vi "SubPanel_DataCollection_Rev11_v13.vi"(0 "DCPowerInformationClusterArray_Input":T6(array[cluster]), 1 "VISAPowerInfoInputArray":T5(array[cluster]), 2 "Run Data SubPanel Input":T4, 3 "RF Block Input Array":T1[](array[typedef]), 4 "Oscilloscope Info Array":T3(array[cluster]) {"vertical coupling" items=["AC", "DC", "Ground"]}, 5 "Plot Color Array":u32[](array[colorbox])=[16711686, 65351, 8978420, 14474240, 16139007, 16752640, 8958719, 16758973, 16777215, 46792, 11992992, 12961221, 16763690, 12600063, 16711835, 2953983, 40796, 13111296, 13352613, 9221011, 12964076, 12819897, 65442, 16776704, 14540253, 16740729, 10658047, 10813344, 16753521, 13413843, 8691115, 10339240, 14401205, 16746704, 7467519, 16775978, 13872558, 11387603, 13354405, 10420227, 13107364, 4060, 35208, 11817216, 7566080, 40796, 7539456, 2837073, 6372186, 7499083, 10648702, 16757152], 6 "New Run?":bool, 7 "error in":errorcluster) -> (20 "DCPowerInformationClusterArray_Output":T6(array[cluster]), 21 "VISAPowerInfoInputOutput":T5(array[cluster]), 22 "Run Data SubPanel Output":T4, 23 "RF Subpanel Output":T1[](array[typedef]), 24 "Oscilloscope Info Array Output":T3(array[cluster]) {"vertical coupling" items=["AC", "DC", "Ground"]}, 25 "Reinitialize?":bool, 26 "Data Was Collected?":bool, 27 "error out":errorcluster)   [LabVIEW 2019]
uses:
  Controls/DataBlockControl.ctl
  Controls/QueueDataControl_V3.ctl
  <vilib>/Utility/file.llb/Write Delimited Spreadsheet (string).vi
  Controls/RFBlockControl.ctl
  <instrlib>/niScope/Controls/niScope vertical coupling.ctl
panel:
  in  "Current Y Min":dbl
  in  "Current Y Max":dbl
  in  "Voltage Y Min":dbl
  in  "Voltage Y Max":dbl
  out "Current Measurements Live":cluster{dbl[], dbl[]}[](graph)
  out "Voltage Measurements Live":cluster{dbl[], dbl[]}[](graph)
  out "RFSourceInfoArray":string[][](array[string])
  out "OscilloscopeInfoArray":string[][](array[string])
  out "Voltage Waveform Array":waveform(dbl)[](graph)
  out "Current Waveform Array":waveform(dbl)[](graph)
  out "DCPowerInfoArray":string[][](array[string])
  out "Current Measurements Total":cluster{dbl[], dbl[]}[](graph)
  out "Voltage Measurements Total":cluster{dbl[], dbl[]}[](graph)
  out "Exiting":bool
  out "Full Run Information":string
  out "Ready For Next Run?":bool
  in  "Next Run":bool
  out "Recording Data":bool
  in  "Record Data Toggle":bool
  out "error of collection":errorcluster
  in  "force exit SubVI":bool
  out "RF Block Parameters Output":T1
  # "Background information (Important)\nThere are three sets of voltage/current graphs\n\nOne is live always and just shows what all the channels look like _______ Waveform Array\n\nOne is live when measuring and shows some duration of the recording _______ Measurements Live\n\nOne shows the entire duration of the run, but it will take a few seconds to compile, just be patient it will populate\n\n\nInstructions (More Important)"
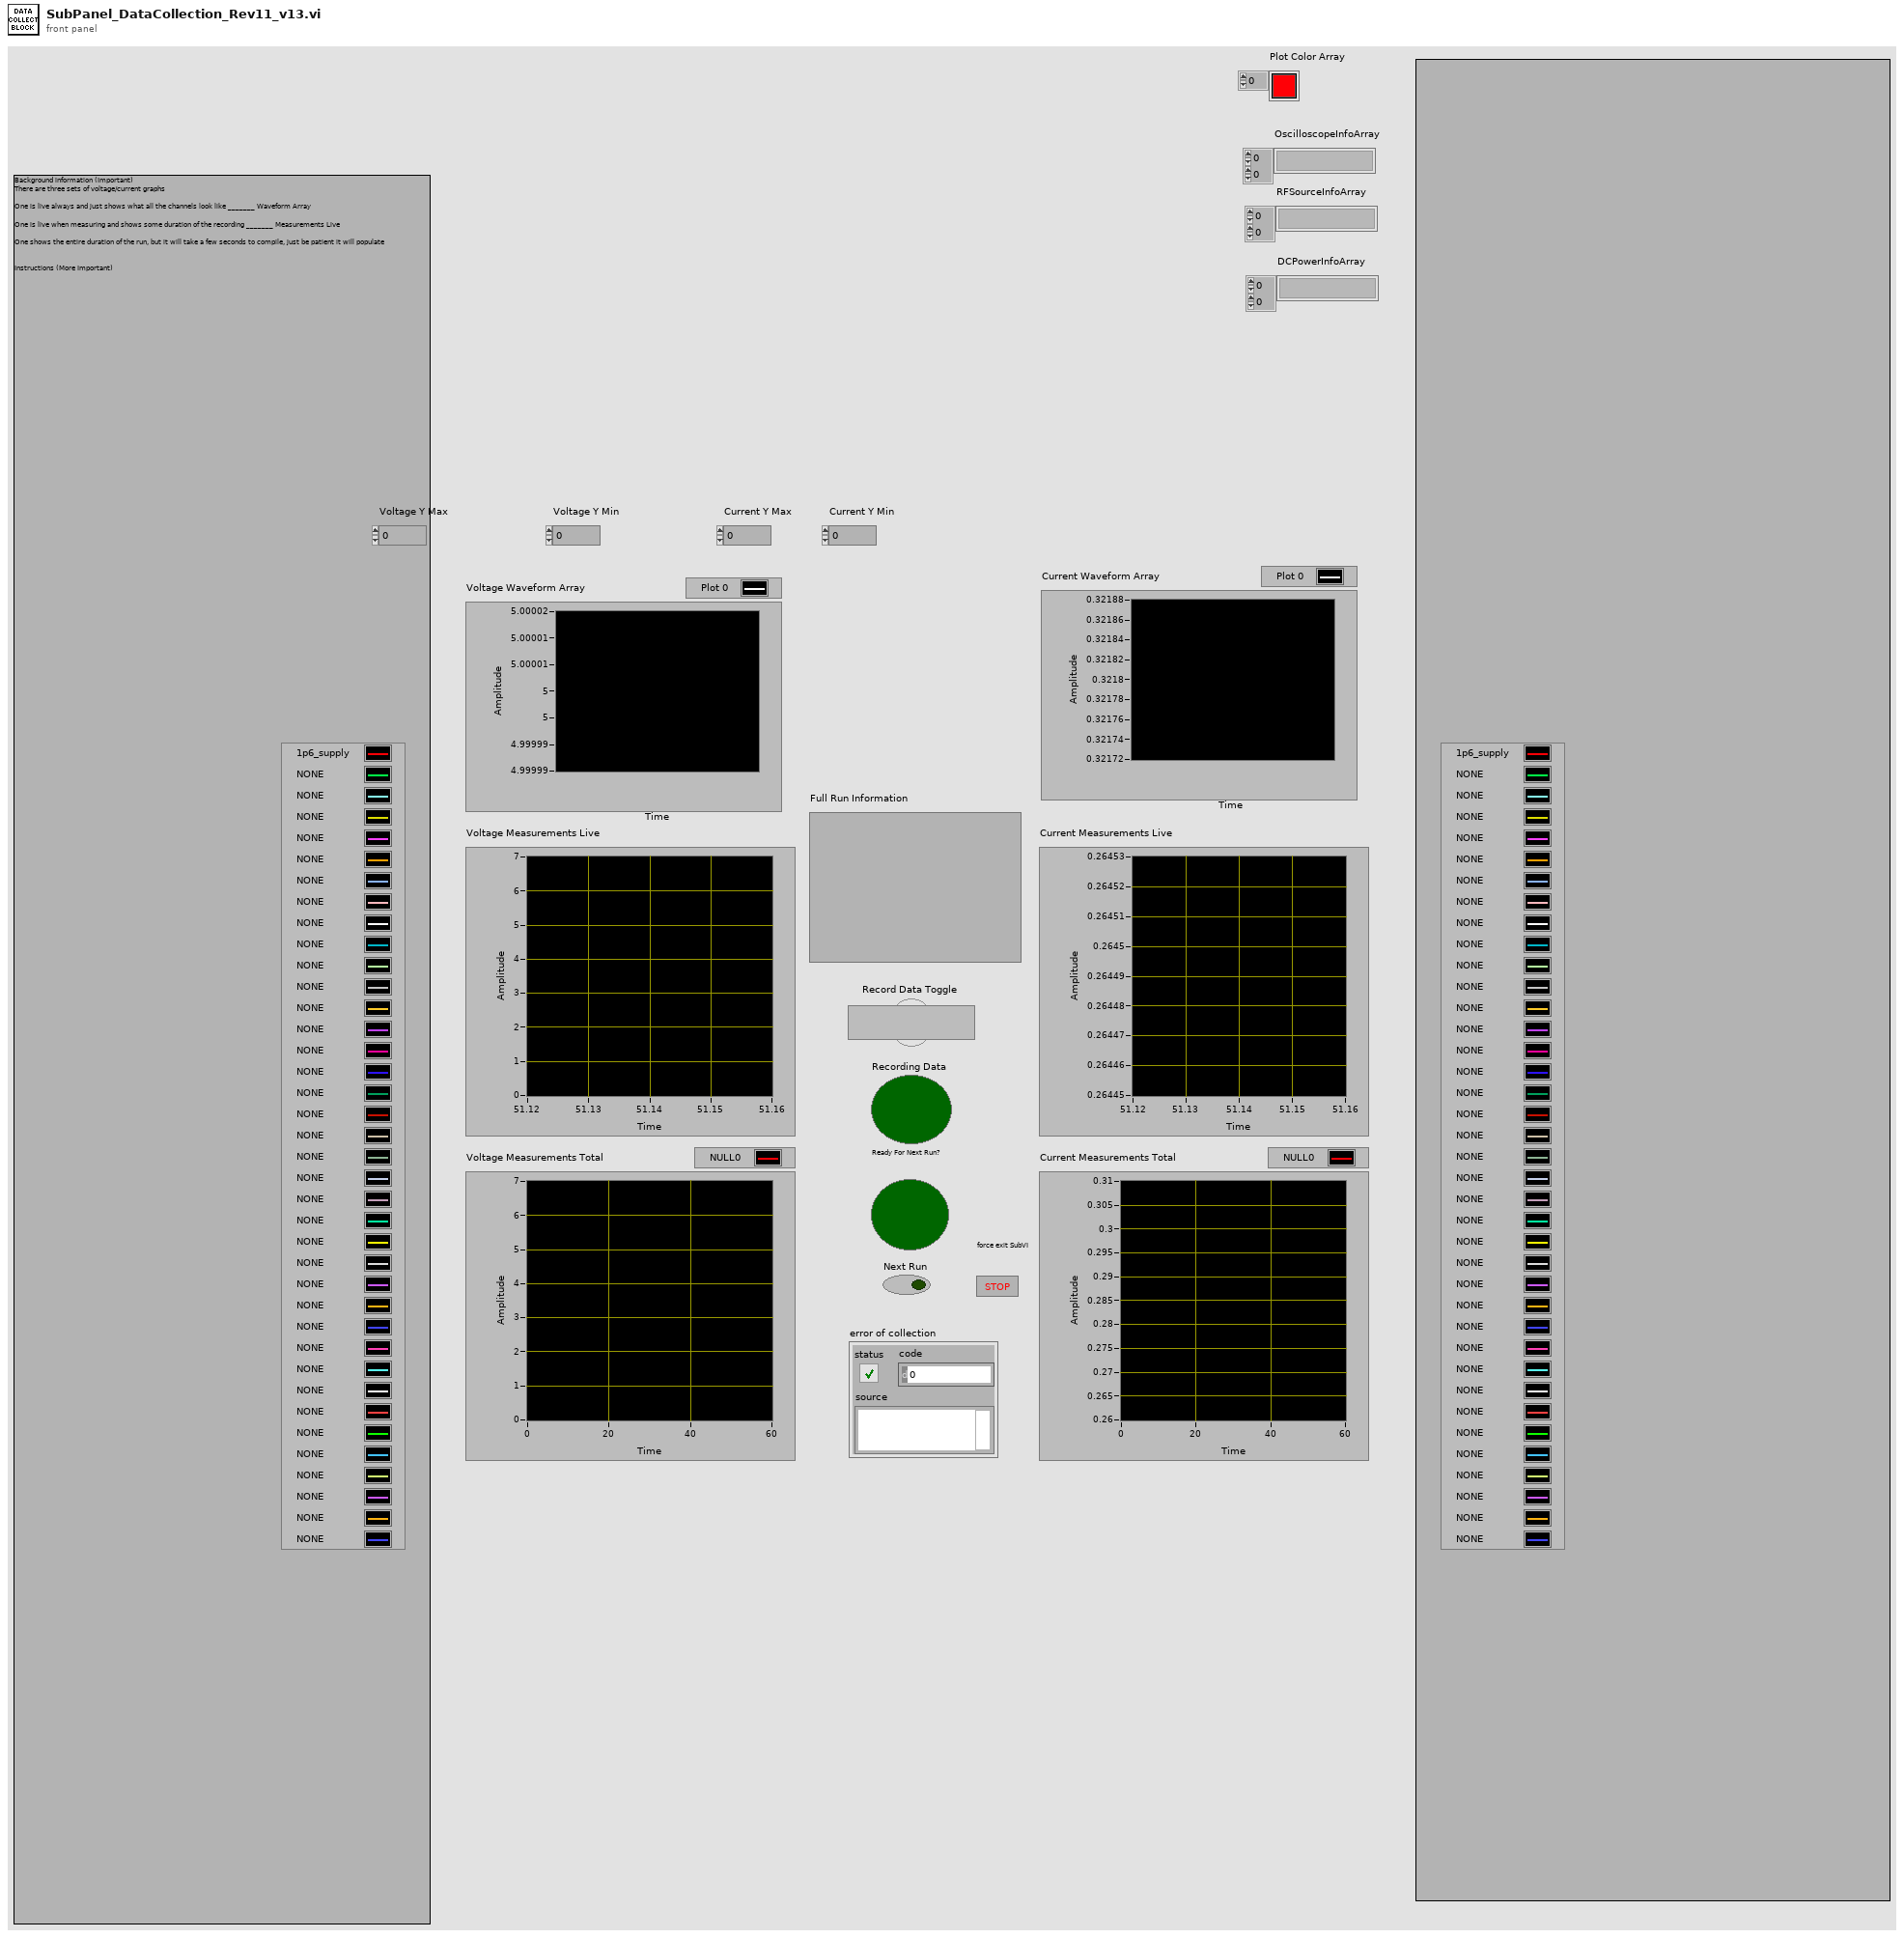
[diagram p1: front panel]
types:
  T1 = typedef "RFBlockControl.ctl" = cluster{"VISA resource name":refnum<visa-resource-name>, "RF Power State In":bool, "Frequency (GHz) Output":dbl, "Power (dBm) Output":dbl, "Instrument Name":string}
  T2 = typedef "niScope vertical coupling.ctl" = i32
  T3 = cluster{"instrument handle out":refnum<k15>, "channel numbers array":string[], "channel names array":string[], "vertical range":dbl, "vertical coupling":T2, "Channel 0 50 ohms?":bool, "50 ohm vertical range (V)":dbl, "min record length":i32, "Actual Sample Rate":dbl}[]
  T4 = typedef "DataBlockControl.ctl" = cluster{"Run Folder Parent Directory":path, "DUT":string, "Ion (ex Kr)":string, "Board Number":string, "Effective LET":string, "Test Type":enum16{"Single Event Latchup", "Single Event Transient", "Single Event Upset"}}
  T5 = cluster{"VISA resource name":refnum<visa-resource-name>, "String List":string, string[], "Input Array (Voltage,Current_Limit)":dbl[], "Input Array (Voltage,Current_Limit)":dbl[], "Channel Names":string[], "read buffer":string}[]
  T6 = cluster{"instrument handle out":refnum<k15>, string, string[], dbl[], string[], "Current Limit Output Array":dbl[], dbl[]}[]
  T7 = typedef "QueueDataControl_V3.ctl" = cluster{"Array of fetched data":dbl[][][], "Channel Names Array":string[], "Voltage Waveform Array":waveform(dbl)[], "Current Waveform Array":waveform(dbl)[], "Resetting Time":timestamp, "Beam Logic":dbl}
  T8 = cluster{"IVI Refnum out":refnum<k15>, string, "voltage level channel 23":dbl, "Channel Name 23":string, "Current Limit":dbl, "Measure Record dt":dbl, string, "Current Threshold Reset Value Array":dbl}[]
  T9 = cluster{"created path array":path[], "DCPowerInformationArrayOutput":cluster{"IVI Refnum out":refnum<k15>, string, "voltage level channel 23":dbl, "Channel Name 23":string, "Current Limit":dbl, "Measure Record dt":dbl, string, "Current Threshold Reset Value Array":dbl}[], string[]}
  T10 = cluster{"Array of fetched data":dbl[][], string, i32[]}
  T11 = enum16{"open", "replace", "create", "open or create", "replace or create", "replace or create with confirmation"}
  T12 = enum16{"Single Event Latchup", "Single Event Transient", "Single Event Upset"}
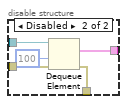
[diagram p4: hidden frame]
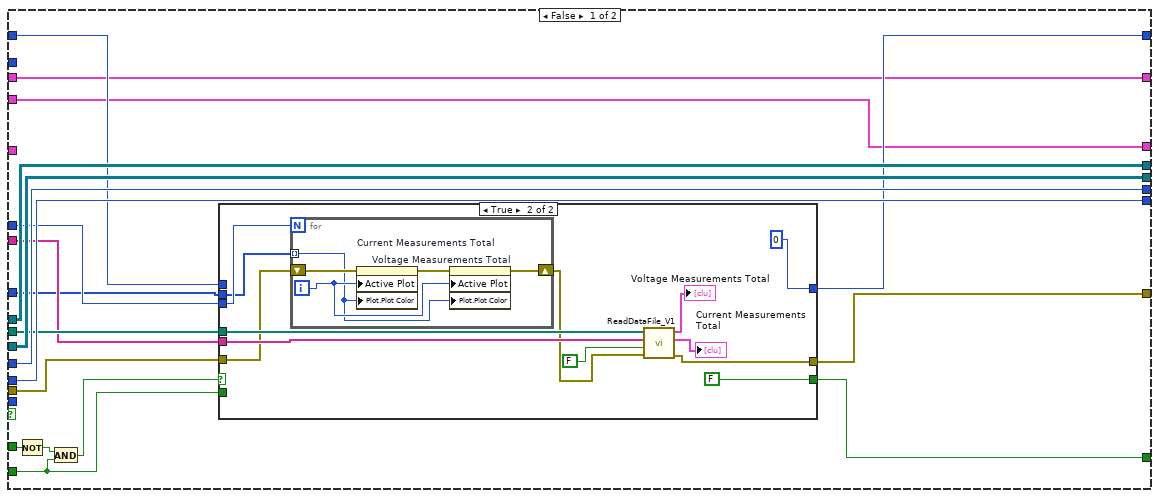
[diagram p5: hidden frame]
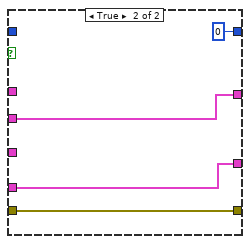
[diagram p7: hidden frame]
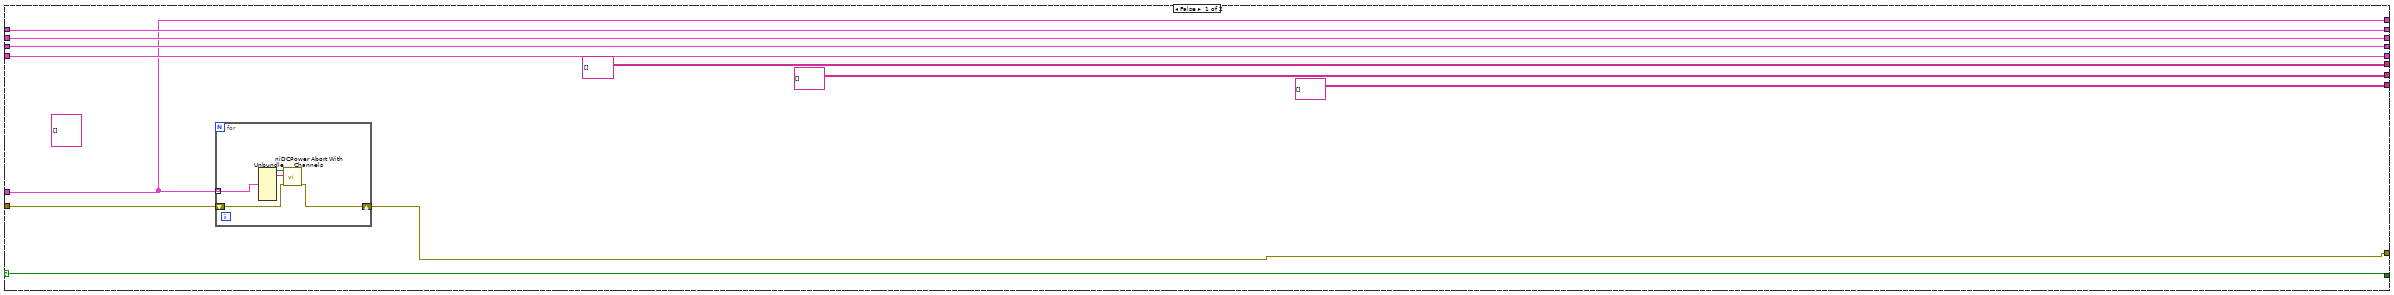
[diagram p8: hidden frame]
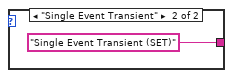
[diagram p9: hidden frame]
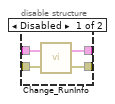
[diagram p13: hidden frame]
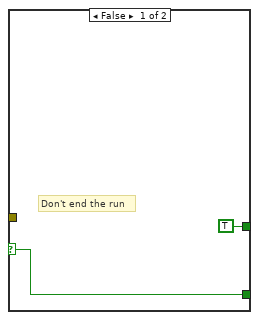
[diagram p16: hidden frame]
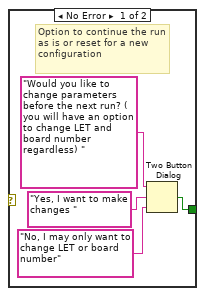
[diagram p17: hidden frame]
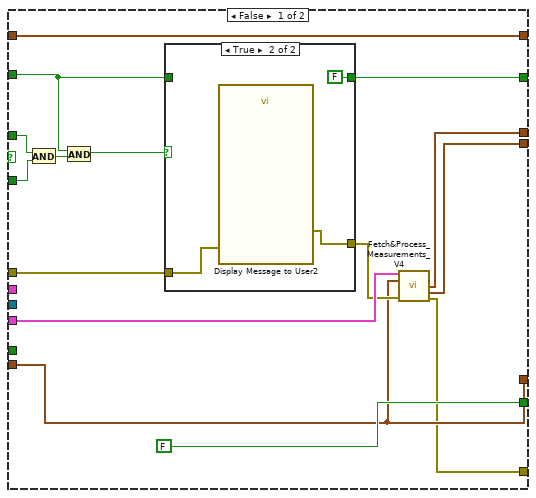
[diagram p19: hidden frame]
diagram:
  w15 = cluster{dbl[], dbl[]}[] [] ("array")
  (unwired) string[] ["Instrument Name", "Channel Name", "Instrument Channel Number", "Voltage (V)", "Current Limit (A)", "Measure Record delta Time (s)"] ("new element/subarray")
  w50 = T7 {"Array of fetched data"=[], "Channel Names Array"=[], "Voltage Waveform Array"=[], "Current Waveform Array"=[], "Resetting Time"=timestamp(0 s since 1904-01-01), "Beam Logic"=0.0} ("DCPower Queue Data Double Array Format")
  (unwired) T7 {"Array of fetched data"=[], "Channel Names Array"=[], "Voltage Waveform Array"=[], "Current Waveform Array"=[], "Resetting Time"=timestamp(0 s since 1904-01-01), "Beam Logic"=0.0} ("DCPower Double Array Queue")
  (unwired) 10000 ("binary file indexor in")
  (unwired) T4 {"Run Folder Parent Directory"=path "", "DUT"="", "Ion (ex Kr)"="", "Board Number"="", "Effective LET"="", "Test Type"=enum."Single Event Latchup"} ("Run Data Configuration")
  # "Need to make a function that will decrease the amount of loops if there are more channels active. Just exponential decay or a X/Y function but need some kind of offset which will probably be experimentally determined"
  # "Initiating the queue"
  # "echoing run information"
  # "Checking if this is a new run. If it is, a new folder is created along with references to a datafile node. If it is not new (i.e. you didn't start recording data because you needed to make a last minute change and pressed forced exit subvi), the previous folder that is theoretically empty (or just has the .txt files is used"
  # "If yes, you go into this subVI"
  # "This is the message at the beginning confirming if you want to make small changes to the program (i.e. LET)"
  # "Parameters from the configuration stage of this program"
  # "Reset the graph that is saving every 10 seconds of data. Every reset the low bound of the ten seconds is"
  # "Need to change to reflect number of channels that are being recorded. Collect this from a parameters file eventually that will be created"
  # "Indicator if the system is ready for another run. Also indicates if data was actually collected"
  # "Resets the system to start recording"
  # "A flag to ensure the warning message shows only once and doesn't lock the system"
  # "Initiating all of the DC Power instruments (doing this here so because we force abort channels in the DCPower setup because buffer overflow issues. Iterating over the instrument array and the active channel list"
  n1 = flat-sequence {
    tunnel: [w90] -> w66
    tunnel: "error in" -> [w80]
    tunnel: [w94] -> w71
    tunnel: "Run Data SubPanel Input" -> [w82]
    frame #0 {
      n2 = disable-structure shown="Enabled" {
        disable-tunnel: w80 -> [w97 w108]
        disable-tunnel: [w106 w108] -> w79
        frame Enabled {
          n3 = property on="Voltage Measurements Live" class="XYGraph (strict)"(error in=w97, "BG Color"=u32 0 ("Plot.Plot Color"), "Plot.Plot Interpolation"=u8 2) -> (error out=w96:errorcluster)  [unwired: 1 in, 1 out]
          n4 = property on="Current Measurements Live" class="XYGraph (strict)"(error in=w96, "BG Color"=u32 0 ("Plot.Plot Color"), "Plot.Plot Interpolation"=u8 2) -> (error out=w95:errorcluster)  [unwired: 1 in, 1 out]
          n5 = property on="Voltage Measurements Total" class="XYGraph (strict)"(error in=w95, "BG Color"=u32 0 ("Plot.Plot Color"), "Plot.Plot Interpolation"=u8 2) -> (error out=w107:errorcluster)  [unwired: 1 in, 1 out]
          n6 = property on="Current Measurements Total" class="XYGraph (strict)"(error in=w107, "BG Color"=u32 0 ("Plot.Plot Color"), "Plot.Plot Interpolation"=u8 2) -> (error out=w106:errorcluster)  [unwired: 1 in, 1 out]
        }
        frame Disabled {
        }
      }
      n7 = local write "Voltage Measurements Total"(cluster{dbl[], dbl[]}[] [] ("Voltage Measurements")) -> ()
      n8 = local write "Current Measurements Total"(cluster{dbl[], dbl[]}[] [] ("Current Measurements")) -> ()
      n9 = local write "Recording Data"(FALSE ("Recording Data")) -> ()
      n10 = local write "Exiting"(FALSE ("Forced Exit")) -> ()
      n11 = call "Convert_RunInfoCluster_2_RunInfoStringList.vi"("error in"=w79, "Run Number"="", "Run Data SubPanel Input"=w82) -> ("error output"=w83:errorcluster, "Run Data Output"=w84:string)
      n12 = call "Display Message to User"("error in (no error)"=w83, "Enable"=TRUE, "Message"=w84) -> ("error out"=w90:errorcluster)  [unwired: 7 in, 1 out]
      n13 = Two Button Dialog(message="Changing the LET?", 1:"No" ("F button name (\"Cancel\")"), 2:"Yes" ("T button name (\"OK\")")) -> (T button?=w94:bool)
    }
  }
  n14 = call "Convert_InstrumentReferenceArray_2_ChannelReferenceArray.vi"("error in (no error)"=w66, "DCPowerInformationClusterArray_Input"="DCPowerInformationClusterArray_Input") -> ("error out"=w65:errorcluster, "DCPowerInformationArrayOutput"=w8:T8)
  n15 = case shown="True" w71 {
    tunnel: "Run Data SubPanel Input" -> [w110 w114]
    tunnel: [w110 w113] -> w24
    tunnel: [w109 w112] -> w67
    tunnel: w65 -> [w109 w111]
    frame False {
    }
    frame True {
      n16 = disable-structure shown="Enabled" {
        disable-tunnel: w114 -> [w118 w120]
        disable-tunnel: [w117 w119] -> w113
        disable-tunnel: [w116 w122] -> w112
        disable-tunnel: w111 -> [w115 w121]
        frame Disabled {
          n17 = call "Change_RunInfo.vi"("error in (no error)"=w115, "Run Data SubPanel in"=w118) -> ("error out"=w116:errorcluster, "Run Data SubPanel out"=w117:T4)
        }
        frame Enabled {
          n18 = call "Change_RunInfo_V2.vi"("error in (no error)"=w121, "Run Data SubPanel in"=w120) -> ("error out"=w122:errorcluster, "Run Data SubPanel out"=w119:T4)
        }
      }
    }
  }
  n19 = Unbundle(w24) -> ("Run Folder Parent Directory"=w68:path)  [unwired: 5 out]
  n20 = List Folder(path=w68, error in=w67) -> (folder names=w69:string[], error out=w53:errorcluster)  [unwired: 2 in, 2 out]
  n21 = Array Size(array=w69) -> (size(s)=w56:i32)
  n22 = case shown="True" "New Run?" {
    selector: "New Run?" -> [w124 w127]
    tunnel: [w125 w129] -> w57
    tunnel: w56 -> [w125 w128]
    tunnel: [w124 w127] -> w55
    tunnel: [w123 w126] -> w54
    tunnel: w53 -> [w123 w126]
    frame False {
    }
    frame True {
      n23 = Increment(x=w128) -> (x+1=w129:i32)
    }
  }
  n24 = Number To Decimal String(number=w57) -> (decimal integer string=w60:string)  [unwired: 1 in]
  n25 = Concatenate Strings("Run_", w60) -> (w23:string)
  n26 = Array Size(array=w8) -> (size(s)=w52:i32)
  n27 = call "InitialFileFolderCreation_V2.vi"("New Run?"=w55, "error in (no error)"=w54, "Run Number"=w23, "Subfolders&NumChannelsRecorded"=w52, "base path"=w68) -> ("error out"=w22:errorcluster, "SupplementalDataFileReferenceObjectArrayWsubfolders"=w63:refnum<file>[][], "DataFileReferenceObjectArrayWsubfolders"=w64:refnum<file>[][], "created path array"=w28:path[])  [unwired: 3 in]
  n28 = call "Convert_RunInfoCluster_2_RunInfoStringList.vi"("error in"=w22, "Run Number"=w23, "Run Data SubPanel Input"=w24) -> ("error output"=w21:errorcluster, "Run Data Output"=→"Full Run Information":string)
  n29 = for {
    shift-right: [w130] -> w4
    shift-left: w21 -> [w132]
    tunnel: "DCPowerInformationClusterArray_Input" -> [w134] mode=indexing
    n30 = Unbundle(w134) -> ("instrument handle out"=w131:refnum<k15>, w133:string)  [unwired: 5 out]
    n31 = call <instrlib>:"niDCPower Initiate With Channels.vi"("error in (no error)"=w132, "channel name"=w133, "instrument handle"=w131) -> ("error out"=w130:errorcluster)  [unwired: 7 in, 1 out]
  }
  n32 = for {
    shift-right: [w137] -> w6
    shift-left: w4 -> [w139]
    tunnel: "Plot Color Array" -> [_] mode=indexing
    i -> [w135]
    w136 = "NONE" ("Plot.Plot Name")
    n33 = property on="Current Measurements Live" class="XYGraph (strict)"(error in=w139, "Active Plot"=w135, "Plot.Plot Name"=w136) -> (error out=w138:errorcluster)  [unwired: 1 in, 1 out]
    n34 = property on="Voltage Measurements Live" class="XYGraph (strict)"(error in=w138, "Active Plot"=w135, "Plot.Plot Name"=w136) -> (error out=w137:errorcluster)  [unwired: 1 in, 1 out]
  }
  n35 = case shown="Error .." w6 {
    selector: w6 -> [w140 _]
    tunnel: [w140 w141] -> w5
    tunnel: w4 -> [_ w141]
    frame No Error {
    }
    frame Error {
    }
  }
  n36 = for {
    tunnel: w8 -> [w144] mode=indexing
    tunnel: [w147] -> w9 mode=indexing
    shift-right: [w143] -> w11
    shift-left: w5 -> [w146]
    tunnel: "Plot Color Array" -> [w142] mode=indexing
    i -> [w148]
    # "Creating Array of Channel Names"
    n37 = Unbundle(w144) -> ("Channel Name 23"=w147:string)  [unwired: 7 out]
    n38 = property on="Current Measurements Live" class="XYGraph (strict)"(error in=w146, "Active Plot"=w148, "Plot.Plot Name"=w147, "Plot.Plot Color"=w142) -> (error out=w145:errorcluster)  [unwired: 1 in, 1 out]
    n39 = property on="Voltage Measurements Live" class="XYGraph (strict)"(error in=w145, "Active Plot"=w148, "Plot.Plot Name"=w147, "Plot.Plot Color"=w142) -> (error out=w143:errorcluster)  [unwired: 1 in, 1 out]
  }
  n40 = disable-structure shown="Enabled" {
    disable-tunnel: w11 -> [w152 w154]
    disable-tunnel: [w151 w154] -> w10
    disable-tunnel: [w150 _] -> w12
    disable-tunnel: w50 -> [w149 _]
    frame Enabled {
      n41 = Obtain Queue(name (unnamed)="DCPowerQueue", element data type=w149, error in (no error)=w152) -> (queue out=w150:refnum<queue>, error out=w151:errorcluster)  [unwired: 2 in, 1 out]
    }
    frame Disabled {
    }
  }
  n42 = Bundle("created path array"=w28, "DCPowerInformationArrayOutput"=w8, w9) -> (w42:T9)  [unwired: 1 in]
  n43 = Array Size(array=w9) -> (size(s)=w14:i32)
  n44 = Get Date/Time In Seconds() -> (seconds since 1Jan1904=w26:timestamp)
  n45 = while {
    shift-right: [w185] -> w32
    shift-left: "DCPowerInformationClusterArray_Input" -> [w185]
    shift-right: [w189] -> w34
    shift-left: "VISAPowerInfoInputArray" -> [w189]
    shift-right: [w188] -> w36
    shift-left: w24 -> [w188]
    shift-right: [w187] -> w38
    shift-left: "RF Block Input Array" -> [w187]
    shift-right: [w186] -> w40
    shift-left: "Oscilloscope Info Array" -> [w186]
    shift-right: [w155] -> w51
    shift-left: w10 -> [w183]
    tunnel: w8 -> [w184]
    shift-right: [w182] -> _
    shift-left: FALSE -> [w179]
    tunnel: w12 -> [w181]
    shift-right: [w165] -> _
    shift-left: FALSE -> [w170]
    tunnel: [w174] -> w75
    shift-right: [w168] -> _
    shift-left: TRUE ("x .and. y?") -> [w169]
    shift-right: [w166] -> _
    shift-left: w26 -> [w167]
    tunnel: [w165] -> w31
    tunnel: w50 -> [w163]
    shift-right: [w160] -> w1
    shift-left: timestamp(0 s since 1904-01-01) ("seconds since 1Jan1904") -> [w159]
    stop <- w164 stop-if-true
    # "If I am going to reset the entire configuration or if we are going up in LET only. True, reset the system. False, don't reset the system"
    n46 = Not(x=w170) -> (.not. x?=w172:bool)
    n47 = And(x="Record Data Toggle", y=w172) -> (x .and. y?=w173:bool)
    "Recording Data" <- w173
    n48 = case shown="True" w173 {
      tunnel: w184 -> [w218 w233]
      tunnel: w183 -> [w216 w240]
      tunnel: [w206 w228] -> w162
      tunnel: [w207 w227] -> w161
      tunnel: w179 -> [_ w238]
      tunnel: [FALSE w239] -> w182
      tunnel: w181 -> [_ w237]
      tunnel: [w205 w236] -> w177
      tunnel: "Record Data Toggle" -> [w213 _]
      tunnel: w170 -> [w214 _]
      tunnel: w169 -> [w209 _]
      tunnel: [w210 TRUE] -> w168
      tunnel: w167 -> [w208 w241]
      tunnel: [w208 w231] -> w166
      tunnel: w163 -> [_ w235]
      tunnel: [w204 w225] -> w160
      tunnel: w159 -> [w204 w224]
      frame False {
        n49 = And(x=w213, y=w214) -> (x .and. y?=w212:bool)
        n50 = And(x=w209, y=w212) -> (x .and. y?=w211:bool)
        n51 = case shown="True" w211 {
          tunnel: [w220 w222] -> w215
          tunnel: w216 -> [w220 w223]
          tunnel: [w219 FALSE] -> w210
          tunnel: w209 -> [w219 _]
          frame False {
          }
          frame True {
            n52 = call "Display Message to User2"("error in (no error)"=w223) -> ("error out"=w222:errorcluster)  [unwired: 9 in, 1 out]
          }
        }
        n53 = call "Fetch&Process_Measurements_V4.vi"("DCPowerInformation_byChannel"=w218, "Initial Time"=w208, "error in (no error)"=w215) -> ("Current Waveform Array"=w206:waveform(dbl)[], "Voltage Waveform Array"=w207:waveform(dbl)[], "error out"=w205:errorcluster)  [unwired: 5 in, 5 out]
      }
      frame True {
        n54 = case shown="True" w238 {
          tunnel: [w243 w249] -> w231
          tunnel: w241 -> [_ w249]
          tunnel: w240 -> [w244 w248]
          tunnel: [w244 w248] -> w232
          tunnel: [TRUE w247] -> w239
          tunnel: w238 -> [_ w247]
          tunnel: [w243 w246] -> w225
          tunnel: w224 -> [_ w246]
          frame False {
            n55 = Get Date/Time In Seconds() -> (seconds since 1Jan1904=w243:timestamp)
          }
          frame True {
          }
        }
        n56 = call "Fetch&Process_Measurements_V4.vi"("DCPowerInformation_byChannel"=w233, "Initial Time"=w231, "error in (no error)"=w232) -> ("Data As dbl Array"=w230:dbl[][][], "Channel Number Array"=w229:string[], "Current Waveform Array"=w228:waveform(dbl)[], "Voltage Waveform Array"=w227:waveform(dbl)[], "error out"=w226:errorcluster)  [unwired: 5 in, 3 out]
        n57 = Bundle(cluster=w235, "Array of fetched data"=w230, "Channel Names Array"=w229) -> (w234:T7)  [unwired: 4 in]
        n58 = Enqueue Element(queue=w237, element=w234, error in (no error)=w226) -> (error out=w236:errorcluster)  [unwired: 1 in, 2 out]
      }
    }
    "Current Waveform Array" <- w162
    "Voltage Waveform Array" <- w161
    n59 = Not(x=w173) -> (.not. x?=w180:bool)
    n60 = And(x=w180, y=w179) -> (x .and. y?=w178:bool)
    n61 = case shown="True" w178 {
      tunnel: w177 -> [w200 w202]
      tunnel: [w201 TRUE] -> w165
      tunnel: w170 -> [w201 _]
      tunnel: [w200 w202] -> w155
      frame False {
      }
      frame True {
      }
    }
    "error of collection" <- w155
    "Ready For Next Run?" <- w165
    n62 = And(x="Next Run", y=w165) -> (x .and. y?=w176:bool)
    n63 = Or(x="force exit SubVI", y=w176) -> (x .or. y?=w157:bool)
    n64 = Or(x=w155, y=w157) -> (x .or. y?=w156:bool)
    n65 = case shown="True" w156 {
      selector: w156 -> [w191 _]
      tunnel: w155 -> [_ w194]
      tunnel: [w191 TRUE] -> w164
      tunnel: [TRUE ("T button?") w192] -> w174
      frame False {
        # "Don't end the run"
      }
      frame True {
        n66 = case shown="Error .." w194 {
          tunnel: [w195 TRUE] -> w192
          frame No Error {
            # "Option to continue the run as is or reset for a new configuration"
            n67 = Two Button Dialog(message="Would you like to change parameters before the next run? ( you will have an option to change LET and board number regardless) ", 1:"No, I may only want to change LET or board number" ("F button name (\"Cancel\")"), 2:"Yes, I want to make changes " ("T button name (\"OK\")")) -> (T button?=w195:bool)
          }
          frame Error {
            # "End the run immediately. There is an error or an immediate issue with the VI"
          }
        }
      }
    }
    "Exiting" <- w164
  }
  "Reinitialize?" <- w75
  n68 = while {
    tunnel: w12 -> [w286]
    shift-right: [w250] -> w47
    shift-left: w10 -> [w285]
    tunnel: w28 -> [w282]
    shift-right: [w275] -> w49
    shift-left: w64 -> [w283]
    shift-right: [w274] -> w48
    shift-left: w63 -> [w281]
    shift-right: [w277] -> _
    shift-left: 0 ("binary file indexor in") -> [w280]
    shift-right: [w276] -> _
    shift-left: 0 ("binary file indexor in") -> [w279]
    tunnel: 1000 ("binary file indexor in") -> [w278]
    tunnel: w9 -> [w284]
    tunnel: w14 -> [w253]
    shift-right: [w263] -> _
    shift-left: FALSE -> [w262]
    shift-right: [w259] -> _
    shift-left: 0 -> [w260]
    shift-right: [w258] -> _
    shift-left: w15 -> [w255]
    shift-right: [w257] -> _
    shift-left: w15 -> [w256]
    tunnel: 251 ("y") -> [w254]
    tunnel: "Plot Color Array" -> [w252]
    stop <- w271 stop-if-true
    # "If recording data is on, there should always be elements in the queue, so I shouldn't have to worry about a state where the \"recording data\" is active but there is no data in the queue, if so, then I'll just have to find an alternative to the OR statement"
    n69 = Get Queue Status(queue=w286, error in (no error)=w285) -> (queue out=w268:refnum<queue>, error out=w269:errorcluster, # elements in queue=w264:i32)  [unwired: 1 in, 5 out]
    n70 = local read "Recording Data"() -> (w261:bool)
    n71 = disable-structure shown="Enabled" {
      disable-tunnel: [w298 w300] -> w270
      disable-tunnel: w269 -> [w297 w302]
      disable-tunnel: w268 -> [w296 w303]
      disable-tunnel: [w295 w299] -> w267
      frame Enabled {
        n72 = Flush Queue(queue=w296, error in (no error)=w297) -> (remaining elements=w295:T7[], error out=w298:errorcluster)  [unwired: 1 out]
      }
      frame Disabled {
        n73 = Dequeue Element(queue=w303, timeout in ms (-1)=100, error in (no error)=w302) -> (element=w299:T7, error out=w300:errorcluster)  [unwired: 2 out]
      }
    }
    n74 = Not Equal To 0?(x=w264) -> (x != 0?=w266:bool)
    n75 = And(x=w266, y=w261) -> (x .and. y?=w265:bool)
    n76 = case shown="True" w265 {
      tunnel: w267 -> [_ w375]
      tunnel: w270 -> [w313 w369]
      tunnel: w284 -> [w314 w362]
      tunnel: w283 -> [w321 w374]
      tunnel: w282 -> [w315 w373]
      tunnel: w281 -> [w322 w372]
      tunnel: w280 -> [w320 w371]
      tunnel: w279 -> [w319 w361]
      tunnel: w278 -> [_ w360]
      tunnel: [w320 w368] -> w277
      tunnel: [w319 w367] -> w276
      tunnel: [w321 w364] -> w275
      tunnel: [w322 w363] -> w274
      tunnel: [w312 w354] -> w251
      tunnel: [w311 TRUE] -> w263
      tunnel: w262 -> [w310 _]
      tunnel: w261 -> [w318 _]
      tunnel: w260 -> [w309 w352]
      tunnel: [w308 w351] -> w259
      tunnel: [w307 w358] -> w258
      tunnel: [w306 w355] -> w257
      tunnel: w256 -> [w306 w350]
      tunnel: w255 -> [w307 w349]
      tunnel: w254 -> [_ w343]
      tunnel: w253 -> [w305 _]
      tunnel: w252 -> [w304 _]
      frame False {
        n77 = Not(x=w318) -> (.not. x?=w317:bool)
        n78 = And(x=w317, y=w310) -> (x .and. y?=w316:bool)
        n79 = case shown="True" w316 {
          tunnel: w315 -> [_ w337]
          tunnel: w314 -> [_ w336]
          tunnel: w313 -> [w325 w329]
          tunnel: [w325 w334] -> w312
          tunnel: [w324 FALSE] -> w311
          tunnel: w310 -> [w324 _]
          tunnel: w309 -> [w323 _]
          tunnel: [w323 0] -> w308
          tunnel: w305 -> [_ w327]
          tunnel: w304 -> [_ w326]
          frame False {
          }
          frame True {
            n80 = for {
              N: w327 -> [_]
              shift-right: [w340] -> w328
              shift-left: w329 -> [w341]
              tunnel: w326 -> [w338] mode=indexing
              i -> [w339]
              n81 = property on="Current Measurements Total" class="XYGraph (strict)"(error in=w341, "Active Plot"=w339, "Plot.Plot Color"=w338) -> (error out=w342:errorcluster)  [unwired: 1 in, 1 out]
              n82 = property on="Voltage Measurements Total" class="XYGraph (strict)"(error in=w342, "Active Plot"=w339, "Plot.Plot Color"=w338) -> (error out=w340:errorcluster)  [unwired: 1 in, 1 out]
            }
            n83 = call "ReadDataFile_V1.vi"("error in (no error)"=w328, "Create CSV files?"=FALSE, "Channel Names Array"=w336, "DataFolder Path"=w337) -> ("error out"=w334:errorcluster, "Current Measurements"=→"Current Measurements Total":cluster{dbl[], dbl[]}[], "Voltage Measurements"=→"Voltage Measurements Total":cluster{dbl[], dbl[]}[])  [unwired: 5 in]
          }
        }
      }
      frame True {
        # "structure where each channel has its own data and supplemental file. Intent for faster data reading speeds in post processing. Probably not since would be i^3, but if we used multiple cores, maybe it would be advantageous"
        n84 = call "FilePathCreation_DCPower_V2.vi"("binary file input reference array 1"=w374, "Channel Name Input array"=w362, "data output directory folder"=w373, "binary file indexor in"=w371, "Reset counter in"=w361, "error in (no error)"=w369, "binary file input reference array 2"=w372, "reset threshold"=w360) -> ("binary file output reference array"=w366:refnum<file>[], "binary file output reference array 2"=w365:refnum<file>[], "binary file indexor out"=w368:i32, "reset counter out"=w367:i32, "error out"=w370:errorcluster)  [unwired: 3 in]
        n85 = for {
          shift-right: [w422] -> w353
          shift-left: w370 -> [w423]
          tunnel: w375 -> [w432]
          tunnel: w365 -> [w429] mode=indexing
          tunnel: w366 -> [w428] mode=indexing
          tunnel: [w427] -> w363 mode=indexing
          tunnel: [w421] -> w364 mode=indexing
          tunnel: [w410] -> w357 mode=indexing
          tunnel: [w409] -> w356 mode=indexing
          i -> [w426]
          n86 = for {
            tunnel: w432 -> [w445] mode=indexing
            tunnel: w426 -> [w442]
            tunnel: [w437] -> w417 mode=concatenating
            tunnel: [w441] -> w431
            tunnel: w429 -> [w440]
            tunnel: w428 -> [w438]
            tunnel: [w438] -> w424
            tunnel: [w440] -> w427
            tunnel: [w439] -> w430 mode=concatenating
            n87 = Unbundle(w445) -> ("Array of fetched data"=w444:dbl[][][], "Channel Names Array"=w443:string[])  [unwired: 4 out]
            n88 = Index Array(array=w443, index=w442) -> (element=w441:string)
            n89 = Index Array(array=w444, index (dim 0)=w442) -> (element=w437:dbl[][])  [unwired: 2 in]
            n90 = Array Size(array=w437) -> (size(s)=w439:i32[])
          }
          n91 = Bundle("Array of fetched data"=w417, w431, w430) -> (w425:T10)  [unwired: 1 in]
          n92 = Index Array(array=w417, index (row)=2) -> (element=w414:dbl[])  [unwired: 1 in]
          n93 = Index Array(array=w417, index (row)=1) -> (element=w415:dbl[])  [unwired: 1 in]
          n94 = Index Array(array=w417, index (row)=0) -> (element=w416:dbl[])  [unwired: 1 in]
          n95 = call "DataFileNode_Entry_V4.vi"("error in (no error)"=w423, "Queued Elements"=w425, "Byte Stream File in"=w424) -> ("error out"=w422:errorcluster, "Byte Stream File out"=w421:refnum<file>)  [unwired: 7 in]
          n96 = for {
            tunnel: [w434] -> w413 mode=indexing if=w433
            tunnel: w416 -> [w434] mode=indexing
            tunnel: [w436] -> w411 mode=indexing if=w433
            tunnel: w415 -> [w436] mode=indexing
            tunnel: [w435] -> w412 mode=indexing if=w433
            tunnel: w414 -> [w435] mode=indexing
            n97 = Not Equal To 0?(x=w434) -> (x != 0?=w433:bool)
          }
          n98 = Bundle(w413, w411) -> (w410:cluster{dbl[], dbl[]})  [unwired: 1 in]
          n99 = Bundle(w413, w412) -> (w409:cluster{dbl[], dbl[]})  [unwired: 1 in]
        }
        n100 = Greater?(x=w352, y=w343) -> (0:w345:bool)
        n101 = Array Size(array=w349) -> (size(s)=w348:i32)
        n102 = Equal?(x=w348, y=0) -> (x = y?=w346:bool)
        n103 = Or(x=w345, y=w346) -> (x .or. y?=w344:bool)
        n104 = case shown="False" w344 {
          tunnel: [w381 w405] -> w358
          tunnel: w349 -> [w385 _]
          tunnel: w357 -> [w384 w405]
          tunnel: w350 -> [w383 _]
          tunnel: w356 -> [w382 w406]
          tunnel: [w380 w406] -> w355
          tunnel: [w379 w408] -> w354
          tunnel: w353 -> [w378 w408]
          tunnel: w352 -> [w377 _]
          tunnel: [w376 0] -> w351
          frame False {
            n105 = for {
              tunnel: w385 -> [w404] mode=indexing
              tunnel: w384 -> [w401] mode=indexing
              tunnel: w383 -> [w398] mode=indexing
              tunnel: w382 -> [w397] mode=indexing
              tunnel: [w388] -> w381 mode=indexing
              tunnel: [w387] -> w380 mode=indexing
              shift-right: [w386] -> w379
              shift-left: w378 -> [w386]
              n106 = Unbundle(w404) -> (w403:dbl[], w402:dbl[])
              n107 = Unbundle(w401) -> (w400:dbl[], w399:dbl[])
              n108 = Unbundle(w398) -> (w396:dbl[], w395:dbl[])
              n109 = Unbundle(w397) -> (w394:dbl[], w393:dbl[])
              n110 = Insert Into Array(array=w396, new element=w394) -> (w391:dbl[])  [unwired: 1 in]
              n111 = Insert Into Array(array=w403, new element=w400) -> (w389:dbl[])  [unwired: 1 in]
              n112 = Insert Into Array(array=w395, new element=w393) -> (w392:dbl[])  [unwired: 1 in]
              n113 = Insert Into Array(array=w402, new element=w399) -> (w390:dbl[])  [unwired: 1 in]
              n114 = Bundle(w391, w392) -> (w387:cluster{dbl[], dbl[]})  [unwired: 1 in]
              n115 = Bundle(w389, w390) -> (w388:cluster{dbl[], dbl[]})  [unwired: 1 in]
            }
            n116 = Increment(x=w377) -> (x+1=w376:i32)
          }
          frame True {
          }
        }
        "Voltage Measurements Live" <- w358
        "Current Measurements Live" <- w355
      }
    }
    n117 = case shown="True" {
      selector: _ -> [_ _]
      tunnel: w251 -> [w287 w294]
      tunnel: [w287 w292] -> w250
      frame False {
      }
      frame True {
        n118 = property on="Voltage Measurements Live" class="XYGraph (strict)"(error in=w294, "YScale.Maximum"="Voltage Y Max", "YScale.Minimum"="Voltage Y Min") -> (error out=w293:errorcluster)  [unwired: 1 in, 1 out]
        n119 = property on="Current Measurements Live" class="XYGraph (strict)"(error in=w293, "YScale.Maximum"="Current Y Max", "YScale.Minimum"="Current Y Min") -> (error out=w292:errorcluster)  [unwired: 1 in, 1 out]
      }
    }
    n120 = local read "Exiting"() -> (w273:bool)
    n121 = Equal To 0?(x=w264) -> (x = 0?=w272:bool)
    n122 = And(x=w272, y=w273) -> (x .and. y?=w271:bool)
  }
  n123 = for {
    tunnel: w49 -> [w450] mode=indexing
    tunnel: w48 -> [w448] mode=indexing
    shift-right: [w446] -> w46
    shift-left: w47 -> [w449]
    n124 = Close File(refnum=w450, error in=w449) -> (error out=w447:errorcluster)  [unwired: 1 out]
    n125 = Close File(refnum=w448, error in=w447) -> (error out=w446:errorcluster)  [unwired: 1 out]
  }
  n126 = Merge Errors(w51, w46) -> (w43:errorcluster)
  n127 = Unbundle(w42) -> ("created path array"=w3:path[])  [unwired: 2 out]
  n128 = case shown="True" w31 {
    selector: w31 -> [w457 w597]
    tunnel: w43 -> [w452 w603]
    tunnel: [w461 w535] -> w41
    tunnel: w40 -> [w461 w602]
    tunnel: [w460 w537] -> w39
    tunnel: w38 -> [w460 w601]
    tunnel: [w459 w523] -> w37
    tunnel: w36 -> [w459 w600]
    tunnel: [w458 w540] -> w35
    tunnel: w34 -> [w458 w599]
    tunnel: [w453 w542] -> w33
    tunnel: w32 -> [w453 w598]
    tunnel: [w457 w597] -> w30
    tunnel: [string[][] [] ("DCPowerInfoArray") w533] -> w29
    tunnel: w3 -> [_ w468]
    tunnel: [string[][] [] ("DCPowerInfoArray") w531] -> w18
    tunnel: [string[][] [] ("DCPowerInfoArray") w525] -> w17
    tunnel: [w451 w470] -> w2
    tunnel: w1 -> [_ w469]
    frame False {
      (unwired) string[][][] []
      n129 = for {
        tunnel: w453 -> [w464] mode=indexing
        shift-right: [w465] -> w451
        shift-left: w452 -> [w466]
        n130 = Unbundle(w464) -> ("instrument handle out"=w463:refnum<k15>, w462:string)  [unwired: 5 out]
        n131 = call <instrlib>:"niDCPower Abort With Channels.vi"("error in (no error)"=w466, "channel name"=w462, "instrument handle"=w463) -> ("error out"=w465:errorcluster)  [unwired: 7 in, 1 out]
      }
    }
    frame True {
      # "This will be indexed eventually"
      n132 = for {
        shift-right: [w696] -> w467
        shift-left: w603 -> [w708]
        tunnel: w598 -> [w699] mode=indexing
        shift-right: [w707] -> w573
        shift-left: w602 -> [w707]
        shift-right: [w706] -> w572
        shift-left: w601 -> [w706]
        shift-right: [w705] -> w571
        shift-left: w600 -> [w705]
        shift-right: [w704] -> w570
        shift-left: w599 -> [w704]
        shift-right: [w703] -> w569
        shift-left: w598 -> [w703]
        shift-right: [w701] -> w574
        shift-left: string[][] [] ("DCPowerInfoArray") -> [w702]
        # "This puts all the instruments together in one output"
        n133 = Unbundle(w699) -> ("instrument handle out"=w710:refnum<k15>, w709:string)  [unwired: 5 out]
        n134 = call <instrlib>:"niDCPower Abort With Channels.vi"("error in (no error)"=w708, "channel name"=w709, "instrument handle"=w710) -> ("error out"=w697:errorcluster)  [unwired: 7 in, 1 out]
        n135 = call "DCPower_ParameterCreation.vi"("error in"=w697, "Precision"="8", "DCPowerInformationByInstrument"=w699) -> ("error out"=w696:errorcluster, "DCPowerInfoArray"=w695:string[][])
        n136 = Insert Into Array(array=w702, index (col)=0 ("disabled index (col)"), new element=w695) -> (w701:string[][])  [unwired: 1 in]
      }
      n137 = Concatenate Strings("Channel Name " ("string")) -> (w586:string)
      n138 = Concatenate Strings("Voltage (V) " ("string")) -> (w588:string)
      n139 = Concatenate Strings("Measure Record delta Time (s) " ("string")) -> (w590:string)
      n140 = Concatenate Strings("Instrument Name " ("string")) -> (w585:string)
      n141 = Concatenate Strings("Instrument Channel Number " ("string")) -> (w587:string)
      n142 = Concatenate Strings("Current Limit (A) " ("string")) -> (w589:string)
      n143 = Build Array(w585, w586, w587, w588, w589, w590) -> (w578:string[])
      n144 = Build Path(base path=w468, name or relative path="DCPOW_Params.csv") -> (appended path=w593:path)
      n145 = Insert Into Array(array=w574, index (col)=0 ("disabled index (col)"), new element=w578) -> (w577:string[][])  [unwired: 1 in]
      n146 = call-poly <vilib>:"Write Delimited Spreadsheet.vi"("file path (dialog if empty)"=w593, "format (%s)"="%s" ("format (%.3f)"), "2D data"=w577, "error in (no error)"=w467, "transpose? (no:F)"=TRUE, "delimiter (\\t)"="," ("delimiter (\\t)")) -> ("error out"=w575:errorcluster)  [unwired: 8 in, 1 out]
      n147 = for {
        shift-right: [w689] -> w555
        shift-left: w575 -> [w689]
        shift-right: [w684] -> w543
        shift-left: w569 -> [w684]
        shift-right: [w685] -> w541
        shift-left: w570 -> [w685]
        shift-right: [w686] -> w539
        shift-left: w571 -> [w686]
        shift-right: [w687] -> w538
        shift-left: w572 -> [w687]
        shift-right: [w688] -> w534
        shift-left: w574 -> [w688]
        tunnel: w573 -> [w683] mode=indexing
        tunnel: [w683] -> w536 mode=indexing
        shift-right: [w652] -> w532
        shift-left: string[][] [] ("DCPowerInfoArray") -> [w658]
        n148 = Unbundle(w683) -> ("instrument handle out"=w682:refnum<k15>, "channel numbers array"=w655:string[], "channel names array"=w656:string[], "vertical range"=w677:dbl, "vertical coupling"=w671:T2, "Channel 0 50 ohms?"=w676:bool, "50 ohm vertical range (V)"=w675:dbl, "min record length"=w670:i32, "Actual Sample Rate"=w669:dbl)
        n149 = Array Size(array=w655) -> (size(s)=w678:i32)
        n150 = Initialize Array(w677, w678) -> (w674:dbl[])
        n151 = Decimal String To Number(string="8") -> (number=w653:i32)  [unwired: 2 in, 1 out]
        n152 = case shown="True" w676 {
          tunnel: w675 -> [_ w692]
          tunnel: w674 -> [w690 w694]
          tunnel: [w690 w691] -> w673
          frame False {
          }
          frame True {
            n153 = Replace Array Subset(array=w694, new element=w692, index=0) -> (w691:dbl[])
          }
        }
        n154 = Number To Fractional String(number=w669, precision (6)=w653) -> (F-format string=w663:string)  [unwired: 2 in]
        n155 = Number To Decimal String(number=w670) -> (decimal integer string=w664:string)  [unwired: 1 in]
        n156 = Concatenate Strings(w682) -> (w680:string)
        n157 = Number To Fractional String(number=w673, precision (6)=w653) -> (F-format string=w672:string[])  [unwired: 2 in]
        n158 = Number To Decimal String(number=w671) -> (decimal integer string=w665:string)  [unwired: 1 in]
        n159 = Array Size(array=w655) -> (size(s)=w681:i32)
        n160 = Initialize Array(w680, w681) -> (w679:string[])
        n161 = Array Size(array=w655) -> (size(s)=w668:i32)
        n162 = Array Size(array=w655) -> (size(s)=w666:i32)
        n163 = Array Size(array=w655) -> (size(s)=w667:i32)
        n164 = Initialize Array(w665, w668) -> (w662:string[])
        n165 = Initialize Array(w663, w666) -> (w660:string[])
        n166 = Initialize Array(w664, w667) -> (w661:string[])
        n167 = Build Array(w679, w656, w655, w672, w662, w661, w660) -> (w657:string[][])
        n168 = Insert Into Array(array=w658, index (col)=0 ("disabled index (col)"), new element=w657) -> (w652:string[][])  [unwired: 1 in]
      }
      n169 = Build Array("Instrument Name " ("string"), "Channel Name" ("element"), "Instrument Channel Number" ("element"), "Vertical Range (V)" ("element"), "Vertical Coupling" ("element"), "Min Record Length" ("element"), "Actual Sample Rate" ("element")) -> (w559:string[])
      n170 = Insert Into Array(array=w532, index (col)=0 ("disabled index (col)"), new element=w559) -> (w552:string[][])  [unwired: 1 in]
      n171 = Build Path(base path=w468, name or relative path="Oscilloscope_Params.csv") -> (appended path=w557:path)
      n172 = call-poly <vilib>:"Write Delimited Spreadsheet.vi"("file path (dialog if empty)"=w557, "format (%s)"="%s" ("format (%.3f)"), "2D data"=w552, "error in (no error)"=w555, "transpose? (no:F)"=TRUE, "delimiter (\\t)"="," ("delimiter (\\t)")) -> ("error out"=w550:errorcluster)  [unwired: 8 in, 1 out]
      n173 = for {
        shift-right: [w634] -> w548
        shift-left: string[][] [] ("DCPowerInfoArray") -> [w635]
        tunnel: w538 -> [w650] mode=indexing
        shift-right: [w619] -> w524
        shift-left: w550 -> [w626]
        shift-right: [w627] -> w531
        shift-left: w532 -> [w627]
        shift-right: [w628] -> w533
        shift-left: w534 -> [w628]
        shift-right: [w629] -> w535
        shift-left: w536 -> [w629]
        shift-right: [w630] -> w537
        shift-left: w538 -> [w630]
        shift-right: [w631] -> w523
        shift-left: w539 -> [w631]
        shift-right: [w632] -> w540
        shift-left: w541 -> [w632]
        shift-right: [w633] -> w542
        shift-left: w543 -> [w633]
        n174 = Unbundle(w650) -> ("VISA resource name"=w649:refnum<visa-resource-name>, "Frequency (GHz) Output"=w643:dbl, "Power (dBm) Output"=w640:dbl)  [unwired: 2 out]
        n175 = Decimal String To Number(string="8") -> (number=w638:i32)  [unwired: 2 in, 1 out]
        n176 = VISA Write(VISA resource name=w649, write buffer="*IDN?", error in (no error)=w626) -> (VISA resource name out=w645:refnum<visa-resource-name>, return count=w647:u32, error out=w651:errorcluster)
        n177 = Number To Fractional String(number=w640, precision (6)=w638) -> (F-format string=w641:string)  [unwired: 2 in]
        n178 = Add(x=w647, y=u32 10) -> (x+y=w644:u32)
        n179 = Number To Fractional String(number=w643, precision (6)=w638) -> (F-format string=w642:string)  [unwired: 2 in]
        n180 = VISA Read(VISA resource name=w645, byte count=w644, error in (no error)=w651) -> (read buffer=w625:string, error out=w620:errorcluster)  [unwired: 2 out]
        n181 = Search and Replace String(replace all?=TRUE ("replace all? (F)"), input string=w625, search string=",", replace string="_" ("replace string (\"\")"), error in=w620) -> (result string=w622:string, error out=w619:errorcluster)  [unwired: 3 in, 2 out]
        n182 = Build Array(w622, w642, w641) -> (w637:string[])
        n183 = Insert Into Array(array=w635, index (col)=0 ("index (row)"), new element=w637) -> (w634:string[][])  [unwired: 1 in]
      }
      n184 = Build Array("Instrument Name", "Frequency (GHz)" ("element"), "Power (dBm)" ("element")) -> (w544:string[])
      n185 = Build Path(base path=w468, name or relative path="RFSource_Params.csv") -> (appended path=w529:path)
      n186 = Insert Into Array(array=w548, index (col)=0 ("disabled index (col)"), new element=w544) -> (w525:string[][])  [unwired: 1 in]
      n187 = call-poly <vilib>:"Write Delimited Spreadsheet.vi"("file path (dialog if empty)"=w529, "format (%s)"="%s" ("format (%.3f)"), "2D data"=w525, "error in (no error)"=w524, "transpose? (no:F)"=TRUE, "delimiter (\\t)"="," ("delimiter (\\t)")) -> ("error out"=w504:errorcluster)  [unwired: 8 in, 1 out]
      n188 = Strip Path(path=w468) -> (name=w522:string)  [unwired: 1 out]
      n189 = Unbundle(w523) -> ("DUT"=w521:string, "Ion (ex Kr)"=w520:string, "Board Number"=w519:string, "Effective LET"=w518:string, "Test Type"=w517:T12)  [unwired: 1 out]
      n190 = case shown="\"Single Event Latchup\", Default" w517 {
        tunnel: ["Single Event Latchup (SEL)" "Single Event Transient (SET)"] -> w516
        frame "Single Event Latchup", Default {
        }
        frame "Single Event Transient" {
        }
      }
      n191 = Build Array("Run Number" ("name"), "DUT" ("element"), "Ion" ("element"), "Board Number" ("element"), "Effective LET" ("element"), "Test Type" ("element")) -> (w515:string[])
      n192 = Build Array(w522, w521, w520, w519, w518, w516) -> (w514:string[])
      n193 = Build Array(w515, w514) -> (w503:string[][])
      n194 = Build Path(base path=w468, name or relative path="RunData_Params.csv") -> (appended path=w509:path)
      n195 = call-poly <vilib>:"Write Delimited Spreadsheet.vi"("file path (dialog if empty)"=w509, "format (%s)"="%s" ("format (%.3f)"), "2D data"=w503, "error in (no error)"=w504, "transpose? (no:F)"=TRUE, "delimiter (\\t)"="," ("delimiter (\\t)")) -> ()  [unwired: 8 in, 2 out]
      n196 = List Folder(path=w468, pattern="*NULL.txt") -> (path out=w487:path, filenames=w488:string[], error out=w489:errorcluster)  [unwired: 2 in, 1 out]
      n197 = for {
        tunnel: [w604] -> w499
        tunnel: w487 -> [w604]
        tunnel: w488 -> [w606] mode=indexing
        shift-right: [w607] -> w490
        shift-left: w489 -> [w608]
        n198 = Build Path(base path=w604, name or relative path=w606) -> (appended path=w605:path)
        n199 = Delete(path (use dialog)=w605, error in=w608) -> (error out=w607:errorcluster)  [unwired: 3 in, 2 out]
      }
      n200 = Get Date/Time String(date format (0)=enum16{"short", "long", "abbreviated"}."short", seconds (now)=w469, want seconds? (F)=TRUE) -> (date string=w493:string, time string=w492:string)
      n201 = Concatenate Strings(w493, "_" ("string"), w492) -> (w494:string)
      n202 = Strip Path(path=w499) -> (name=w485:string)  [unwired: 1 out]
      n203 = Build Path(base path=w499, name or relative path="BeginRecordTimeStamp.txt") -> (appended path=w500:path)
      n204 = Concatenate Strings(w485, "_DCPOWER_COPYFOLDER" ("name or relative path")) -> (w486:string)
      n205 = Open/Create/Replace File(file path (use dialog)=w500, error in=w490, operation (0:open)=T11."open or create", access (0:read/write)=enum16{"read/write", "read-only", "write-only"}."read/write") -> (refnum out=w495:refnum<file>, error out=w491:errorcluster)  [unwired: 2 in, 1 out]
      n206 = Build Path(base path=w499, name or relative path=w486) -> (appended path=w479:path)
      n207 = Write to Text File(file (use dialog)=w495, text=w494, error in=w491) -> (refnum out=w497:refnum<file>, error out=w496:errorcluster)  [unwired: 1 in, 1 out]
      n208 = Close File(refnum=w497, error in=w496) -> (error out=w498:errorcluster)  [unwired: 1 out]
      n209 = Create Folder(path (use dialog)=w479, error in=w498) -> (created path=w483:path, error out=w480:errorcluster)  [unwired: 1 in, 1 out]
      n210 = List Folder(path=w499, error in=w480) -> (path out=w481:path, filenames=w482:string[], error out=w484:errorcluster)  [unwired: 2 in, 1 out]
      n211 = for {
        tunnel: w481 -> [w614]
        tunnel: w482 -> [w613] mode=indexing
        tunnel: w483 -> [w609]
        shift-right: [w616] -> w470
        shift-left: w484 -> [w610]
        tunnel: [w609] -> _
        n212 = Build Path(base path=w614, name or relative path=w613) -> (appended path=w611:path)
        n213 = Build Path(base path=w609, name or relative path=w613) -> (appended path=w612:path)
        n214 = Copy(8:w610, 9:TRUE ("overwrite (F)"), 10:w612, 11:w611) -> (0:w616:errorcluster)  [unwired: 1 in, 2 out]
      }
    }
  }
  "DCPowerInformationClusterArray_Output" <- w33
  "VISAPowerInfoInputOutput" <- w35
  "Run Data SubPanel Output" <- w37
  "Oscilloscope Info Array Output" <- w41
  "Data Was Collected?" <- w30
  "DCPowerInfoArray" <- w29
  "OscilloscopeInfoArray" <- w18
  "RFSourceInfoArray" <- w17
  "RF Subpanel Output" <- w39
  "error out" <- w2
